vi "Noise-Create (Inverse Filtered).vi"(0 "Noise In":T5, 5 "Level In":T3, 7 "Filter In":T1 {"Stages"."IIR Filter"."Forward Coefficients" format="%.4f"; "Stages"."IIR Filter"."Reverse Coefficients" format="%.4f"}, 9 "Fs (Hz)":dbl, 11 "error in (no error)":errorcluster, 12 "Token length (s)":dbl=3.14365) -> (4 "Noise Out":T5, 6 "Level Out":T3, 8 "Filter Out":T1 {"Stages"."IIR Filter"."Forward Coefficients" format="%.4f"; "Stages"."IIR Filter"."Reverse Coefficients" format="%.4f"}, 10 "InvFilter Noise":dbl[](array[numeric]), 15 "error out":errorcluster)   [LabVIEW 2020]
uses:
  Noise Params.ctl
  Controls/Level XCtl/Level Data.ctl
  Controls/Level XCtl/Level Units.ctl
  Controls/Advanced Filter XCtl/Filter Data.ctl
  Filter VIs/Filter-Bandwidth Units.ctl
  epl-cal-vi-lib/Inverse Filter VIs/InvFilt-Params.ctl
  Controls/Advanced Filter XCtl/Advanced Filter XCtl.xctl
  Controls/Level XCtl/Level XCtl.xctl
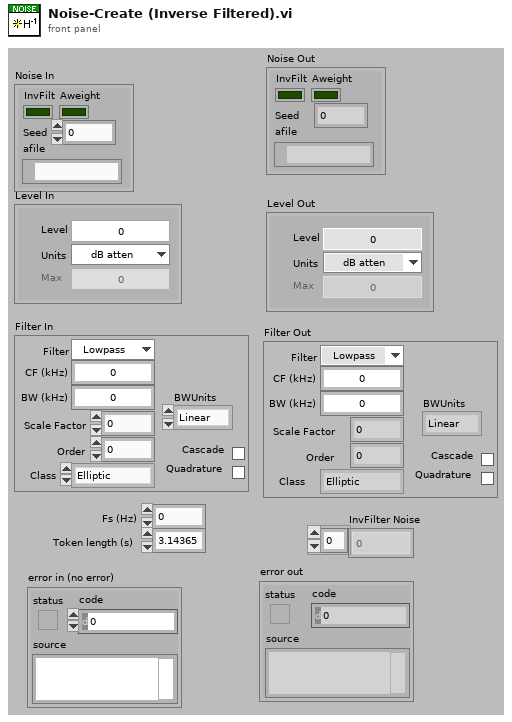
[diagram p1: front panel]
types:
  T1 = typedef "Advanced Filter XCtl.xctl/Filter Data.ctl" = cluster{"Type":enum16{"Lowpass", "Highpass", "Bandpass", "Bandstop", "OFF"}, "CF (kHz)":dbl, "BW (kHz)":dbl, "Cascade":bool, "Quadrature":bool, "Scale Factor":dbl, "Stages":cluster{"IIR Filter":cluster{"filter structure":enum32{"IIR 2nd Order", "IIR 4th Order"}, "Reverse Coefficients":dbl[], "Forward Coefficients":dbl[]}, "State":dbl[]}[], "Class":enum16{"Elliptic", "Butterworth"}, "Order":i32, "BWUnits":T2}
  T2 = typedef "Filter-Bandwidth Units.ctl" = enum16{"Linear", "Octaves", "Min-Max"}
  T3 = typedef "Level XCtl.xctl/Level Data.ctl" = cluster{"Level":dbl, "Units":T4, "Max":dbl, "Multiplier":dbl, "Cal File":path, "Cal":cluster{"Freq (Hz)":dbl[], "Mag (dB SPL)":dbl[], "Phase (deg)":dbl[]}}
  T4 = typedef "Level Units.ctl" = enum16{"dB atten", "dB SPL", "dB re 1 Vrms", "dB V/Hz½", "mW", "dB HL", "Volts", "dB mW"}
  T5 = typedef "Noise Params.ctl" = cluster{"InvFilt":bool, "Noise":dbl[], "CurPt":i32, "Aweight":bool, "Seed":i32, "afile":path}
  T6 = typedef "InvFilt-Params.ctl" = cluster{"Min Frequency (Hz)":dbl, "Max Frequency (Hz)":dbl, "Length (points)":i32, "Sampling rate (Hz)":dbl, "Delay (ms)":dbl, "Linear phase":bool}
  T7 = enum16{"Lowpass", "Highpass", "Bandpass", "Bandstop", "OFF"}
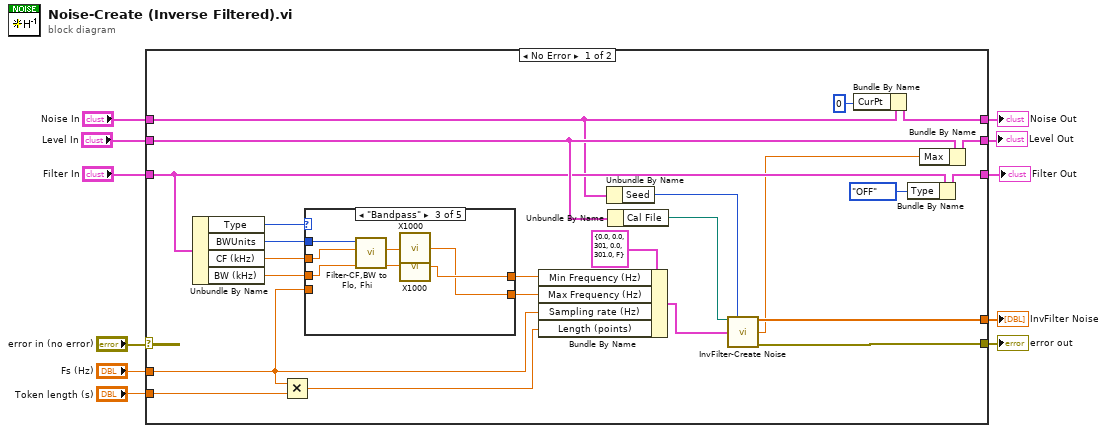
[diagram p0: block diagram]
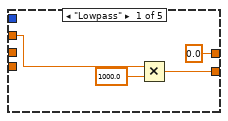
[diagram p2: hidden frame]
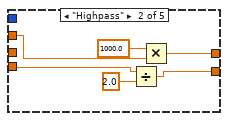
[diagram p3: hidden frame]
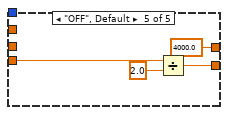
[diagram p5: hidden frame]
diagram:
  n1 = case shown="No Error" "error in (no error)" {
    selector: "error in (no error)" -> [_ w60]
    tunnel: [w23 w60] -> w10
    tunnel: "Noise In" -> [w14 w59]
    tunnel: "Fs (Hz)" -> [w26 _]
    tunnel: "Token length (s)" -> [w28 _]
    tunnel: [w25 w59] -> w4
    tunnel: [w22 _] -> w7
    tunnel: "Filter In" -> [w19 w57]
    tunnel: "Level In" -> [w20 w58]
    tunnel: [w16 w58] -> w2
    tunnel: [w18 w57] -> w1
    frame No Error {
      n2 = Unbundle By Name(w19) -> ("Type"=w33:T7, "BWUnits"=w12:T2, "CF (kHz)"=w30:dbl, "BW (kHz)"=w29:dbl)
      n3 = Multiply(x=w26, y=w28) -> (x*y=w27:dbl)
      n4 = case shown="\"Bandpass\"" w33 {
        tunnel: [0.0 w41 w47 _ 4000.0] -> w32
        tunnel: [w37 w43 w46 _ w55] -> w31
        tunnel: w26 -> [_ w44 _ _ w54]
        tunnel: w30 -> [w38 w42 w51 _ _]
        tunnel: w29 -> [_ _ w50 _ _]
        tunnel: w12 -> [_ _ w52 _ _]
        frame "Lowpass" {
          n5 = Multiply(x=w38, y=1000.0) -> (x*y=w37:dbl)
        }
        frame "Highpass" {
          n6 = Divide(x=w44, y=2.0) -> (x/y=w43:dbl)
          n7 = Multiply(x=1000.0, y=w42) -> (x*y=w41:dbl)
        }
        frame "Bandpass" {
          n8 = call "Filter-CF,BW to Flo, Fhi.vi"("BW"=w50, "CF (kHz)"=w51, "BWUnits"=w52) -> ("Fmin"=w48:dbl, "Fmax"=w49:dbl)  [unwired: 7 in]
          n9 = call "X1000.vi"("X"=w49) -> ("X/1000"=w46:dbl)
          n10 = call "X1000.vi"("X"=w48) -> ("X/1000"=w47:dbl)
        }
        frame "Bandstop" {
        }
        frame "OFF", Default {
          n11 = Divide(x=w54, y=2.0) -> (x/y=w55:dbl)
        }
      }
      n12 = Bundle By Name(cluster=T6 {"Min Frequency (Hz)"=0.0, "Max Frequency (Hz)"=0.0, "Length (points)"=301, "Sampling rate (Hz)"=0.0, "Delay (ms)"=301.0, "Linear phase"=FALSE} ("InvFilt Params"), "Min Frequency (Hz)"=w32, "Max Frequency (Hz)"=w31, "Sampling rate (Hz)"=w26, "Length (points)"=w27) -> (w35:T6)
      n13 = Unbundle By Name(w14) -> ("Seed"=w13:i32)
      n14 = Unbundle By Name(w20) -> ("Cal File"=w21:path)
      n15 = call "InvFilter-Create Noise.vi"("Calibration File"=w21, "seed"=w13, "InvFilt Params"=w35) -> ("InvFilter Noise"=w22:dbl[], "Max Level"=w15:dbl, "error out"=w23:errorcluster)  [unwired: 9 in, 1 out]
      n16 = Bundle By Name(cluster=w14, "CurPt"=0 ("Waveform.Noise.CurPt")) -> (w25:T5)
      n17 = Bundle By Name(cluster=w19, "Type"=T7."OFF" ("Filter.Type")) -> (w18:T1)
      n18 = Bundle By Name(cluster=w20, "Max"=w15) -> (w16:T3)
    }
    frame Error {
    }
  }
  "error out" <- w10
  "InvFilter Noise" <- w7
  "Noise Out" <- w4
  "Level Out" <- w2
  "Filter Out" <- w1
